vi "CmdExe.Run Multiple Utilities.vi"(8 "error in (no error)":errorcluster, 9 "Show Cmd Window":bool=TRUE, 10 "Wait til Complete":bool=TRUE, 11 "Util Folder":path=path "C:/MTE/Startup") -> (0 "error out":errorcluster, 3 "Util List":path[](array[path]))   [LabVIEW 2019]
panel:
  in  "Types":string[](array[string])=["*.exe", "*.bat"]
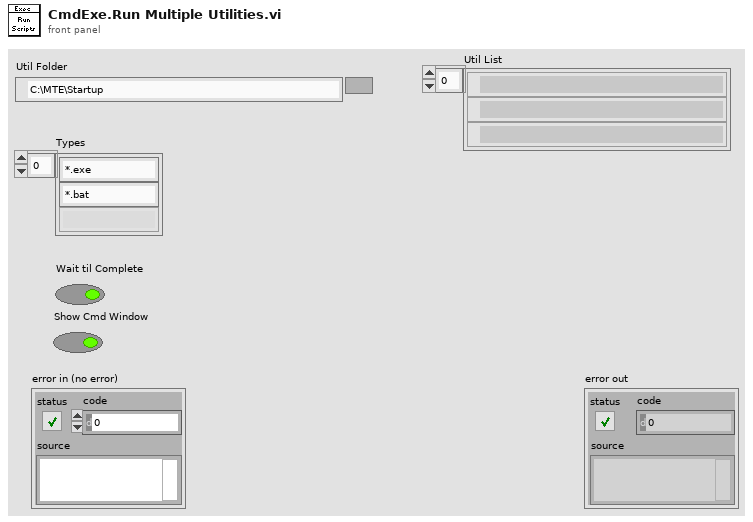
[diagram p1: front panel]
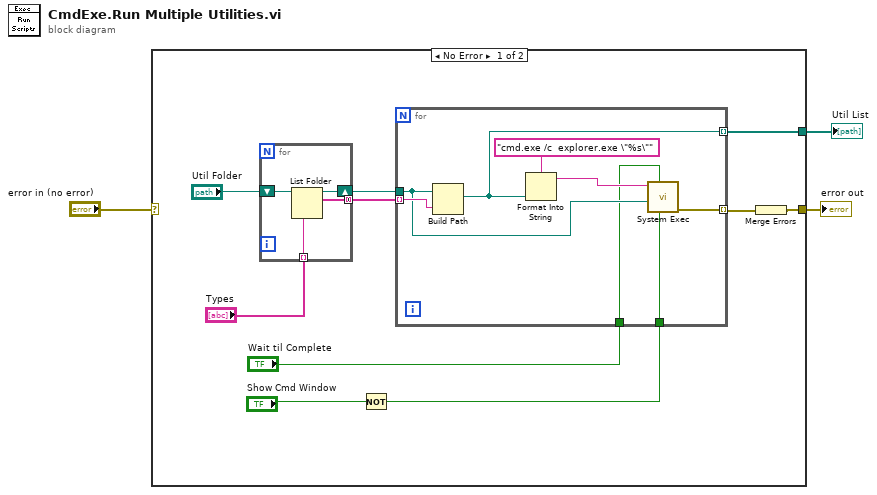
[diagram p0: block diagram]
diagram:
  n1 = case shown="No Error" "error in (no error)" {
    selector: "error in (no error)" -> [_ w26]
    tunnel: [w9 w26] -> w3
    tunnel: [w8 _] -> w2
    frame No Error {
      n2 = for {
        tunnel: [w15] -> w11 mode=concatenating
        shift-right: [w16] -> w12
        shift-left: "Util Folder" -> [w17]
        tunnel: "Types" -> [w14] mode=indexing
        n3 = List Folder(path=w17, pattern=w14) -> (path out=w16:path, filenames=w15:string[])  [unwired: 2 in, 2 out]
      }
      n4 = Not(x="Show Cmd Window") -> (.not. x?=w5:bool)
      n5 = for {
        tunnel: w12 -> [w24]
        tunnel: w11 -> [w25] mode=indexing
        tunnel: [w21] -> w10 mode=indexing
        tunnel: [w20] -> w8 mode=indexing
        tunnel: w5 -> [w19]
        tunnel: "Wait til Complete" -> [w18]
        n6 = Build Path(base path=w24, name or relative path=w25) -> (appended path=w20:path)
        n7 = Format Into String(format string="cmd.exe /c  explorer.exe \"%s\"", w20) -> (resulting string=w22:string)  [unwired: 2 in, 1 out]
        n8 = call <vilib>:"System Exec.vi"("run minimized? (F)"=w19, "wait until completion? (T)"=w18, "working directory"=w24, "command line"=w22) -> ("error out"=w21:errorcluster)  [unwired: 4 in, 3 out]
      }
      n9 = Merge Errors(w10) -> (w9:errorcluster)
    }
    frame Error {
    }
  }
  "error out" <- w3
  "Util List" <- w2
